vi "Destroy_Tag.vi"(8 "error in (no error)":errorcluster, 11 "tag handle":i32) -> (0 "error out":errorcluster, 3 "error code":i32)   [LabVIEW 2019]
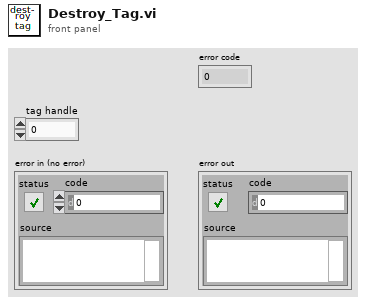
[diagram p1: front panel]
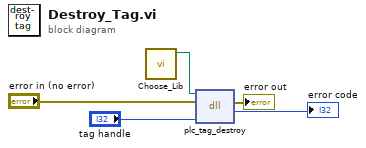
[diagram p0: block diagram]
diagram:
  n1 = call "Choose_Lib.vi"() -> ("appended path"=w1:path)  [unwired: 11 in]
  n2 = dll-call lib="home/dbowden/Desktop/libplctag-master/build/bin_dist/libplctag.so" fn="plc_tag_destroy"(path in=w1, error in="error in (no error)", "tag"="tag handle") -> (error out=→"error out":errorcluster, "return type"=→"error code":i32)  [unwired: 2 in, 1 out]
